vi "array_broadcasting.vi"(1 "broad_array":dbl[][](array[numeric]), 2 "Array":dbl[][](array[numeric])) -> (0 "sum()":dbl[][](array[numeric]))   [LabVIEW 2020]
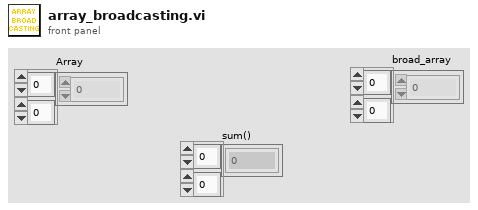
[diagram p1: front panel]
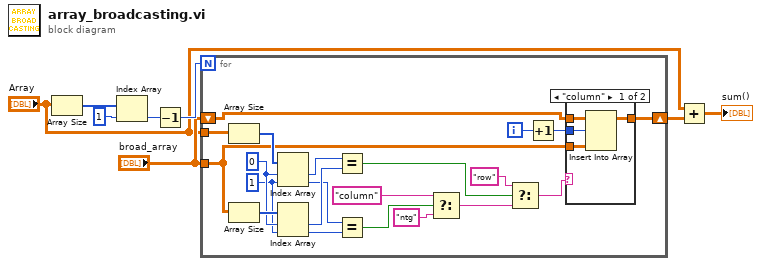
[diagram p0: block diagram]
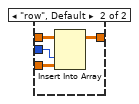
[diagram p2: hidden frame]
diagram:
  n1 = Array Size(array="Array") -> (size(s)=w8:i32[])
  n2 = Index Array(array=w8, index=1) -> (element=w6:i32)
  n3 = Decrement(x=w6) -> (x-1=w5:i32)
  n4 = for {
    N: w5 -> [_]
    tunnel: "broad_array" -> [w9]
    shift-right: [w10] -> w3
    shift-left: "broad_array" -> [w11]
    tunnel: "Array" -> [w29]
    i -> [w13]
    w25 = 1 ("index")
    w26 = 0 ("index")
    n5 = Array Size(array=w29) -> (size(s)=w28:i32[])
    n6 = Array Size(array=w9) -> (size(s)=w27:i32[])
    n7 = Index Array(array=w28, index #1=w26, index #2=w25) -> (element #1=w24:i32, element #2=w20:i32)
    n8 = Index Array(array=w27, index #1=w26, index #2=w25) -> (element #1=w23:i32, element #2=w21:i32)
    n9 = Equal?(x=w24, y=w23) -> (x = y?=w22:bool)
    n10 = Equal?(x=w20, y=w21) -> (x = y?=w19:bool)
    n11 = Select(t="column", s=w19, f="ntg") -> (s? t:f=w16:string)
    n12 = Select(t="row", s=w22, f=w16) -> (s? t:f=w14:string)
    n13 = Increment(x=w13) -> (x+1=w12:i32)
    n14 = case shown="\"column\"" w14 {
      tunnel: w12 -> [w30 w34]
      tunnel: w11 -> [w33 w37]
      tunnel: [w31 w36] -> w10
      tunnel: w9 -> [w32 w35]
      frame "column" {
        n15 = Insert Into Array(array=w33, index (row)=w30, new element=w32) -> (w31:dbl[][])  [unwired: 1 in]
      }
      frame "row", Default {
        n16 = Insert Into Array(array=w37, index (col)=w34, new element=w35) -> (w36:dbl[][])  [unwired: 1 in]
      }
    }
  }
  n17 = Add(x="Array", y=w3) -> (x+y=→"sum()":dbl[][])
